vi "Untitled 5.vi"   [LabVIEW 2011]
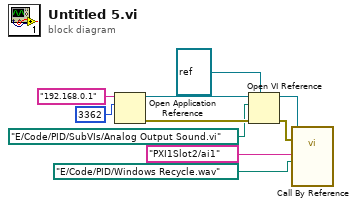
[diagram p0: block diagram]
diagram:
  n1 = Open Application Reference(10:u16 3362 ("port number or service name (3363)"), 11:"192.168.0.1" ("machine name (\"\":  open local reference)")) -> (0:w5:errorcluster, 3:w3:refnum<vi>)  [unwired: 2 in]
  n2 = Open VI Reference(type specifier VI Refnum (for type only)=refnum<vi> refnum, application reference (local)=w3, vi path=path "E:/Code/PID/SubVIs/Analog Output Sound.vi", error in (no error)=w5) -> (vi reference=w9:refnum<vi>, error out=w8:errorcluster)  [unwired: 2 in]
  n3 = call-by-ref "?"(reference=w9, error in=w8, "Sound File"=path "E:/Code/PID/Windows Recycle.wav" ("path"), "physical channels"=tag "PXI1Slot2/ai1") -> ()  [unwired: 10 in, 2 out]
